vi "Plik_auto_nazwa.vi"(6 "Nazwa in":string="DATA", 8 "error in (no error)":errorcluster, 11 "path in":path=path "D:/Marek/Documents/LabVIEW PiWDP instrukcje/Pliki VI/Ćwiczenie 12/Main_maszyna.vi") -> (0 "error out":errorcluster, 3 "path out":path)   [LabVIEW 2013]
doc: "Use this template to build a VI to use as a subVI."
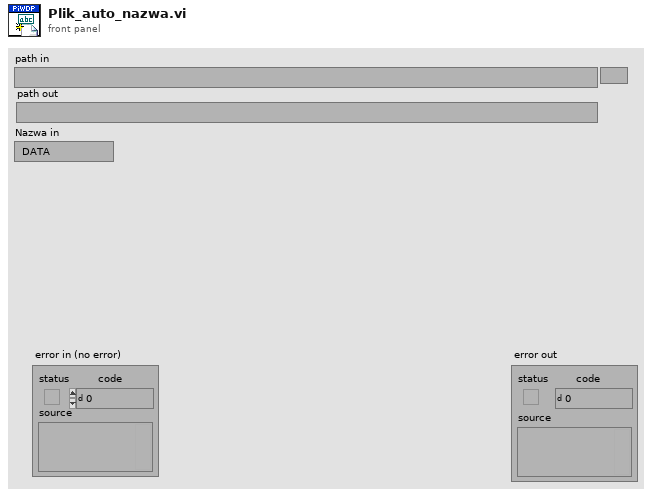
[diagram p1: front panel]
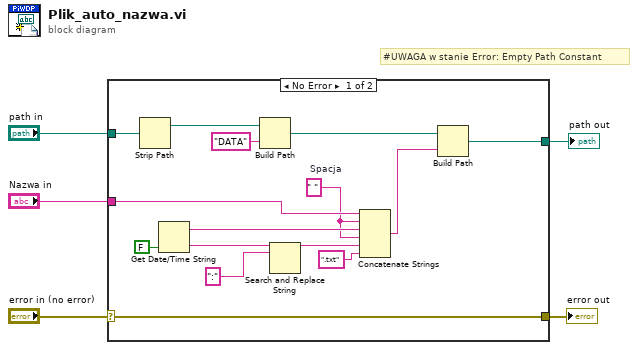
[diagram p0: block diagram]
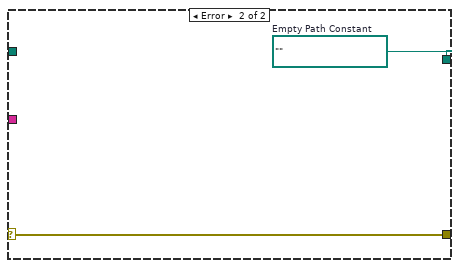
[diagram p2: hidden frame]
diagram:
  # "#UWAGA w stanie Error: Empty Path Constant"
  n1 = case shown="No Error" "error in (no error)" {
    selector: "error in (no error)" -> [w19 w22]
    tunnel: [w19 w22] -> w4
    tunnel: "path in" -> [w18 _]
    tunnel: [w15 w21] -> w2
    tunnel: "Nazwa in" -> [w14 _]
    frame No Error {
      w11 = " "  # Spacja
      n2 = Strip Path(path=w18) -> (stripped path=w17:path)  [unwired: 1 out]
      n3 = Get Date/Time String(want seconds? (F)=FALSE) -> (date string=w12:string, time string=w8:string)  [unwired: 2 in]
      n4 = Build Path(base path=w17, name or relative path="DATA") -> (appended path=w16:path)
      n5 = Search and Replace String(input string=w8, search string=":") -> (result string=w7:string)  [unwired: 6 in, 3 out]
      n6 = Concatenate Strings "Concatenate Strings"(w14, w11, w12, w11, w7, ".txt" ("string")) -> (w13:string)
      n7 = Build Path(base path=w16, name or relative path=w13) -> (appended path=w15:path)
    }
    frame Error {
      w21 = path ""  # Empty Path Constant
    }
  }
  "error out" <- w4
  "path out" <- w2
